vi "Get BrotherNode.vi"(8 "error in (no error)":errorcluster caption="错误输入（无错误）", 11 "PanelLinkNode 输入":refnum<class "PanelLinkNode.lvclass"> caption="DNL_LabVIEW Object in") -> (0 "error out":errorcluster caption="错误输出", 2 "BrotherNode*":refnum<data-value>, 3 "PanelLinkNode 输出":refnum<class "PanelLinkNode.lvclass"> caption="DNL_LabVIEW Object out")   [LabVIEW 2016, in "PanelLinkNode.lvclass"]
uses:
  PanelLinkNode.lvclass
  PanelLinkNode.lvclass/PanelLinkNode.ctl
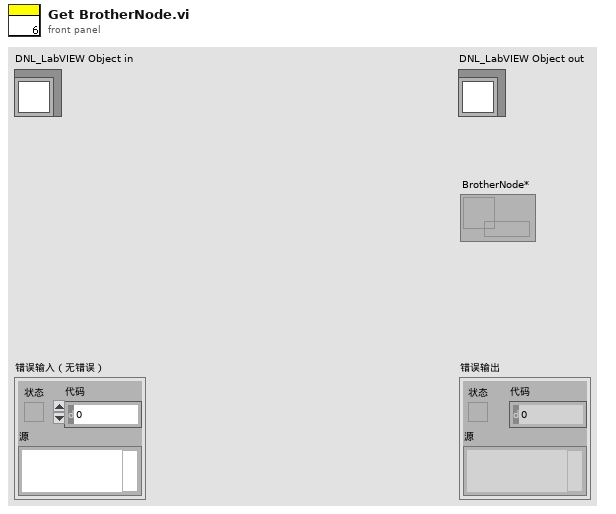
[diagram p1: front panel]
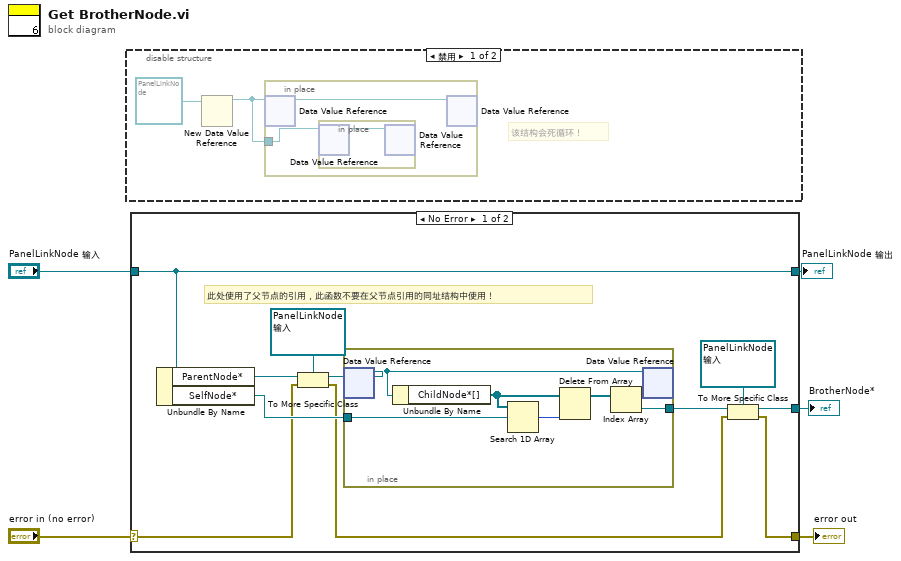
[diagram p0: block diagram]
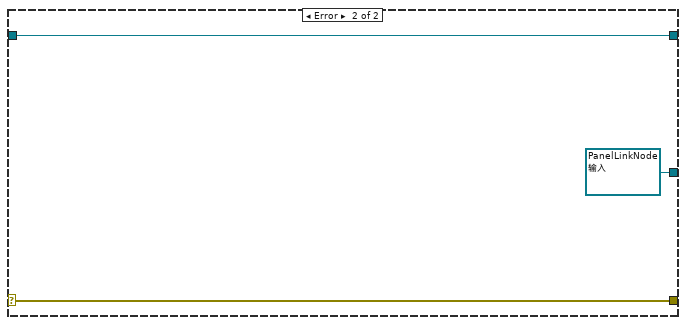
[diagram p3: hidden frame]
diagram:
  n1 = disable-structure shown="禁用" {
    frame Disabled {
      # "该结构会死循环！"
      n2 = New Data Value Reference(data value=refnum<class "PanelLinkNode.lvclass"> refnum ("PanelLinkNode.lvclass")) -> (data value reference=w6:refnum<data-value>)  [unwired: 1 in, 1 out]
      n3 = in-place {
        in-place-border: w6 -> [w9]
        n4 = in-place-dvr #1(w6) -> (w8:refnum<class "PanelLinkNode.lvclass">)  [unwired: 1 out]
        n5 = in-place {
          n6 = in-place-dvr #2(w9) -> (w10:refnum<class "PanelLinkNode.lvclass">)  [unwired: 1 out]
          n7 = in-place-dvr #2(w10) -> ()  [unwired: 2 out]
        }
        n8 = in-place-dvr #1(w8) -> ()  [unwired: 2 out]
      }
    }
    frame Enabled {
    }
  }
  n9 = case shown="No Error" "error in (no error)" {
    selector: "error in (no error)" -> [w13 w30]
    tunnel: [w11 w30] -> w4
    tunnel: [w21 w29] -> w2
    tunnel: "PanelLinkNode 输入" -> [w21 w29]
    tunnel: [w14 refnum<data-value> refnum ("数据值引用")] -> w1
    frame No Error {
      # "此处使用了父节点的引用，此函数不要在父节点引用的同址结构中使用！"
      n10 = Unbundle By Name(w21) -> ("ParentNode*"=w20:refnum<data-value>, "SelfNode*"=w17:refnum<data-value>)
      n11 = To More Specific Class(target class=refnum<data-value> refnum ("数据值引用"), reference=w20, error in=w13) -> (specific class reference=w18:refnum<data-value>, error out=w12:errorcluster)
      n12 = in-place {
        in-place-border: w17 -> [w27]
        in-place-border: [w23] -> w15
        n13 = in-place-dvr #3(w18) -> (w22:refnum<class "PanelLinkNode.lvclass">)  [unwired: 1 out]
        n14 = Unbundle By Name(w22) -> ("ChildNode*[]"=w25:refnum<data-value>[])
        n15 = Search 1D Array(1D array=w25, element=w27) -> (index of element=w26:i32)  [unwired: 1 in]
        n16 = Delete From Array(array=w25, index=w26) -> (array with subset deleted=w24:refnum<data-value>[])  [unwired: 1 in, 1 out]
        n17 = Index Array(array=w24) -> (element=w23:refnum<data-value>)  [unwired: 1 in]
        n18 = in-place-dvr #3(w22) -> ()  [unwired: 2 out]
      }
      n19 = To More Specific Class(target class=refnum<data-value> refnum ("数据值引用"), reference=w15, error in=w12) -> (specific class reference=w14:refnum<data-value>, error out=w11:errorcluster)
    }
    frame Error {
    }
  }
  "error out" <- w4
  "PanelLinkNode 输出" <- w2
  "BrotherNode*" <- w1
